vi "original_trigger.vi"(3 "last sync value":bool, 4 "counter in":i16, 5 "sync minimum high":i16=1000) -> (0 "DIO stored in shift registar":bool, 1 "counter out":i16, 2 "trigger out":bool)   [LabVIEW 2010]
uses:
  <vilib>/eio/EIONode/EIONode.xnode
  <vilib>/rvi/eio/nirviEIOImplementation/nirviEIOImplementation.xnode
  <vilib>/rvi/eio/common/nirviEmuClasses.ctl
  <vilib>/rvi/eio/common/nirviEmuTemplateMethod_noerrors.vi
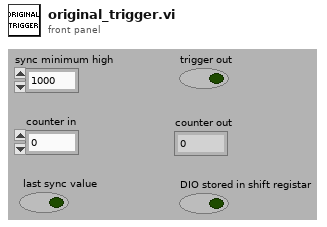
[diagram p1: front panel]
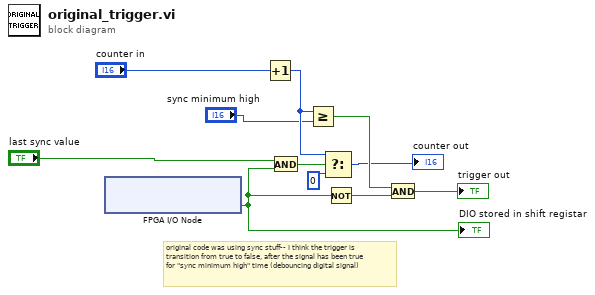
[diagram p0: block diagram]
diagram:
  # "original code was using sync stuff-- I think the trigger is \ntransition from true to false, after the signal has been true \nfor \"sync minimum high\" time (debouncing digital signal)"
  n1 = xnode "FPGA I/O Node"() -> ("Connector0/DIO6"=w11:bool)  [unwired: 1 in, 1 out]
  "DIO stored in shift registar" <- w11
  n2 = Increment(x="counter in") -> (x+1=w7:i16)
  n3 = And(x="last sync value", y=w11) -> (x .and. y?=w3:bool)
  n4 = Greater Or Equal?(x=w7, y="sync minimum high") -> (x >= y?=w9:bool)
  n5 = Select(t=w7, s=w3, f=i16 0) -> (s? t:f=→"counter out":i16)
  n6 = Not(x=w11) -> (.not. x?=w8:bool)
  n7 = And(x=w9, y=w8) -> (x .and. y?=→"trigger out":bool)
